vi "Limelight.vi"() -> ()   [LabVIEW 2018]
uses:
  5bda4818-5db7-4a37-94fe-e126cb2a47b4.vi
  65baa005-36a5-4b5c-ad00-e7831b38fc40.vi
  ffe1e7bf-722c-4abf-afb3-08bbb05ce56e.vi
  cfa8c977-f46c-4ebb-8e7e-f5b631340d2e.vi
  20f04a56-a653-4d81-a16d-e2cce2d6ced9.vi
  75f726a3-edf9-46da-8158-0b1851abcaf1.vi
  6606baff-e82b-4fed-8c44-0260f9793549.vi
  <vilib>/Array/Sort 2D Array - Pop Stack.vi
  <vilib>/Array/Sort 2D Array - Push Stack.vi
  <vilib>/Rock Robotics/Network Tables/NT Read Numeric Array.vi
panel:
  out "Height":dbl
  out "Center":dbl
  out "Degrees Off":dbl
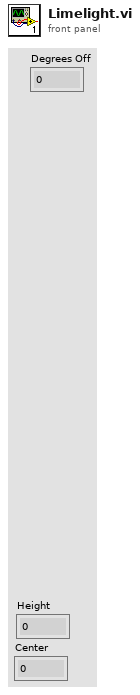
[diagram p1: front panel]
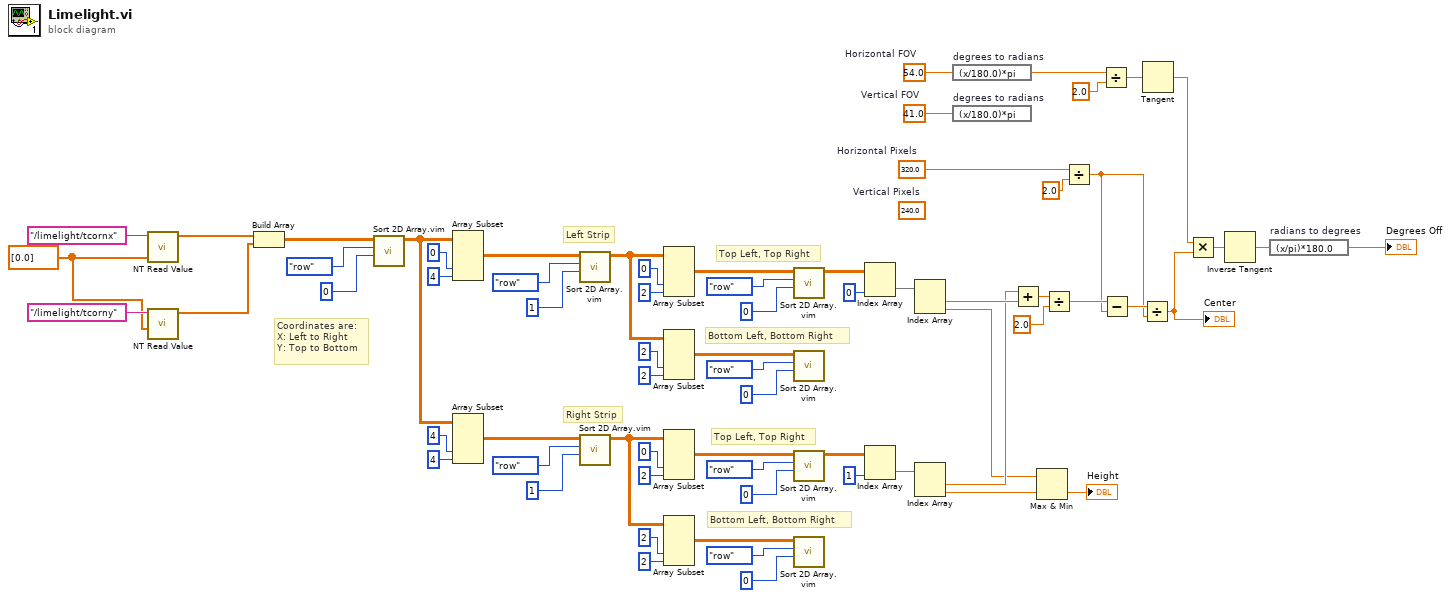
[diagram p0: block diagram]
diagram:
  (unwired) 240.0  # Vertical Pixels
  w5 = 320.0  # Horizontal Pixels
  w14 = 41.0  # Vertical FOV
  w17 = 54.0  # Horizontal FOV
  w65 = dbl[] [0.0] ("Default Value")
  # "Coordinates are:\nX: Left to Right\nY: Top to Bottom"
  # "Top Left, Top Right"
  # "Bottom Left, Bottom Right"
  # "Top Left, Top Right"
  # "Bottom Left, Bottom Right"
  # "Right Strip"
  # "Left Strip"
  n1 = call-poly <vilib>:"NT Read Value.vi"("Default Value"=w65, "Name"="/limelight/tcornx") -> ("Numeric Array"=w67:dbl[])  [unwired: 8 in, 1 out]
  n2 = call-poly <vilib>:"NT Read Value.vi"("Default Value"=w65, "Name"="/limelight/tcorny") -> ("Numeric Array"=w66:dbl[])  [unwired: 8 in, 1 out]
  n3 = Build Array(w67, w66) -> (w62:dbl[][])
  n4 = call "Sort 2D Array.vim"("index"=0, "dimension to index (column)"=enum16{"column", "row"}."row", "2D array"=w62) -> ("sorted 2D array"=w57:dbl[][])  [unwired: 7 in, 1 out]
  n5 = Array Subset(array=w57, index (col)=0 ("index"), length (col)=4 ("index")) -> (w54:dbl[][])  [unwired: 2 in]
  n6 = Array Subset(array=w57, index (col)=4 ("index"), length (col)=4 ("index")) -> (w51:dbl[][])  [unwired: 2 in]
  n7 = call "Sort 2D Array.vim"("index"=1, "dimension to index (column)"=enum16{"column", "row"}."row", "2D array"=w54) -> ("sorted 2D array"=w46:dbl[][])  [unwired: 7 in, 1 out]
  n8 = call "Sort 2D Array.vim"("index"=1, "dimension to index (column)"=enum16{"column", "row"}."row", "2D array"=w51) -> ("sorted 2D array"=w41:dbl[][])  [unwired: 7 in, 1 out]
  n9 = Array Subset(array=w46, index (col)=0 ("index"), length (col)=2 ("index")) -> (w38:dbl[][])  [unwired: 2 in]
  n10 = Array Subset(array=w46, index (col)=2 ("index"), length (col)=2 ("index")) -> (w35:dbl[][])  [unwired: 2 in]
  n11 = Array Subset(array=w41, index (col)=0 ("index"), length (col)=2 ("index")) -> (w30:dbl[][])  [unwired: 2 in]
  n12 = Array Subset(array=w41, index (col)=2 ("index"), length (col)=2 ("index")) -> (w29:dbl[][])  [unwired: 2 in]
  n13 = call "Sort 2D Array.vim"("index"=0, "dimension to index (column)"=enum16{"column", "row"}."row", "2D array"=w38) -> ("sorted 2D array"=w26:dbl[][])  [unwired: 7 in, 1 out]
  n14 = call "Sort 2D Array.vim"("index"=0, "dimension to index (column)"=enum16{"column", "row"}."row", "2D array"=w35) -> ()  [unwired: 7 in, 2 out]
  n15 = call "Sort 2D Array.vim"("index"=0, "dimension to index (column)"=enum16{"column", "row"}."row", "2D array"=w30) -> ("sorted 2D array"=w25:dbl[][])  [unwired: 7 in, 1 out]
  n16 = call "Sort 2D Array.vim"("index"=0, "dimension to index (column)"=enum16{"column", "row"}."row", "2D array"=w29) -> ()  [unwired: 7 in, 2 out]
  n17 = Index Array(array=w26, index (col)=0 ("disabled index (col)")) -> (element=w24:dbl[])  [unwired: 1 in]
  n18 = Index Array(array=w25, index (col)=1 ("disabled index (col)")) -> (element=w23:dbl[])  [unwired: 1 in]
  n19 = Index Array(array=w24) -> (element #1=w22:dbl, element #2=w20:dbl)  [unwired: 2 in]
  n20 = Index Array(array=w23) -> (element #1=w21:dbl, element #2=w19:dbl)  [unwired: 2 in]
  n21 = expression code="(x/180.0)*pi" "degrees to radians"(w17) -> (w15:dbl)
  n22 = expression code="(x/180.0)*pi" "degrees to radians"(w14) -> ()  [unwired: 1 out]
  n23 = Add(x=w21, y=w22) -> (x+y=w9:dbl)
  n24 = Max & Min(x=w20, y=w19) -> (min(x,y)=→"Height":dbl)  [unwired: 1 out]
  n25 = Divide(x=w9, y=2.0 ("x+y")) -> (x/y=w7:dbl)
  n26 = Divide(x=w5, y=2.0) -> (x/y=w2:dbl)
  n27 = Divide(x=w15, y=2.0) -> (x/y=w13:dbl)
  n28 = Subtract(x=w7, y=w2) -> (x-y=w6:dbl)
  n29 = Divide(x=w6, y=w2) -> (x/y=w3:dbl)
  "Center" <- w3
  n30 = Tangent(1:w13) -> (0:w12:dbl)
  n31 = Multiply(x=w12, y=w3) -> (x*y=w11:dbl)
  n32 = Inverse Tangent(1:w11) -> (0:w10:dbl)
  n33 = expression code="(x/pi)*180.0" "radians to degrees"(w10) -> (→"Degrees Off":dbl)
